vi "Drive y-axis x feet.vi"(11 "Feet":dbl) -> ()   [LabVIEW 2017]
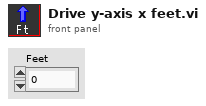
[diagram p1: front panel]
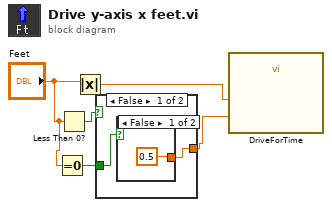
[diagram p0: block diagram]
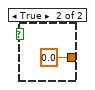
[diagram p2: hidden frame]
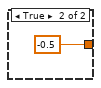
[diagram p3: hidden frame]
diagram:
  n1 = Equal To 0?(x="Feet") -> (x = 0?=w1:bool)
  n2 = Less Than 0?(x="Feet") -> (x < 0?=w4:bool)
  n3 = Absolute Value(x="Feet") -> (abs(x)=w5:dbl)
  n4 = case shown="False" w4 {
    tunnel: [w6 -0.5] -> w3
    tunnel: w1 -> [w7 _]
    frame False {
      n5 = case shown="False" w7 {
        tunnel: [0.5 0.0] -> w6
        frame False {
        }
        frame True {
        }
      }
    }
    frame True {
    }
  }
  n6 = call "DriveForTime.vi"("Time(s)"=w5, "Y"=w3) -> ()  [unwired: 10 in]
